vi "TestSuite_SQLiteOverallOperationCheck.vi"() -> ()   [LabVIEW 2014, in "TableLogger_SQLite_Actor.lvlib" / "TableLogger_SQLite_Actor.lvclass"]
uses:
  TableLogger_SQLite_Actor.lvclass
  TableLogger_Actor/TableLoggerConfig.ctl
  TableLogger_Actor/TableLoggerTypes.ctl
  TableLogger_Actor/TableLoggerBackupConfig.ctl
  <vilib>/addons/_JKI Toolkits/Caraya/classes/Test Suite/Test Suite.lvclass
  TableLogger_Actor/TableLogger_Actor.lvlib
panel:
  out "error out":errorcluster
  in  "error in (no error)":errorcluster
  # "Test Suite to Check overall operation of SQLite Logger"
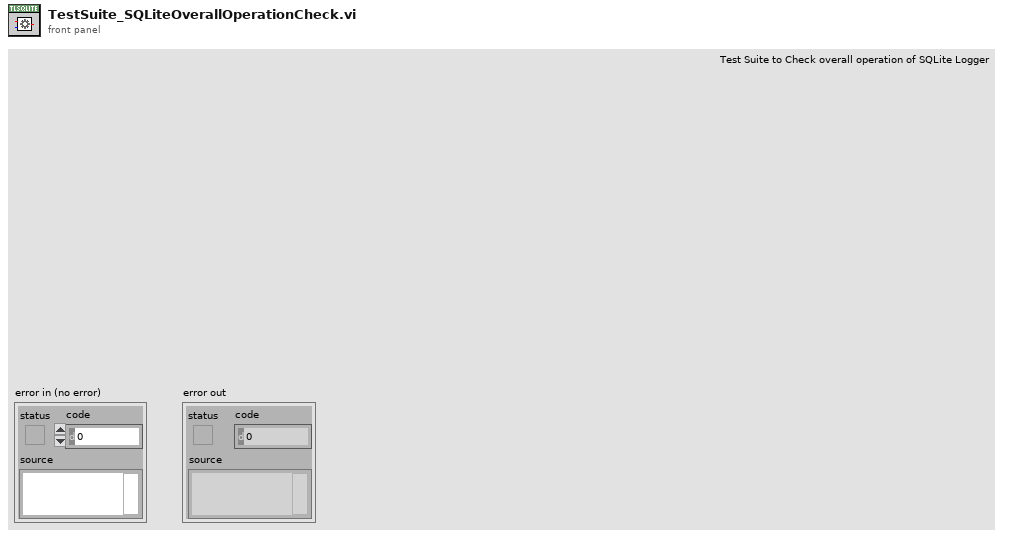
[diagram p1: front panel]
types:
  T1 = typedef "TableLogger_Actor.lvlib/TableLoggerConfig.ctl" = cluster{"TableLogger":T2, "DB File Path":path, "DB Backup Config":T3}
  T2 = typedef "TableLogger_Actor.lvlib/TableLoggerTypes.ctl" = enum16{"CSV Logger", "SQLite Logger"}
  T3 = typedef "TableLogger_Actor.lvlib/TableLoggerBackupConfig.ctl" = cluster{"Directory":path, "UTC Time Format":bool, "On Launch":bool, "Interval (Hours)":dbl, "Size Multiples (Bytes)":i32}
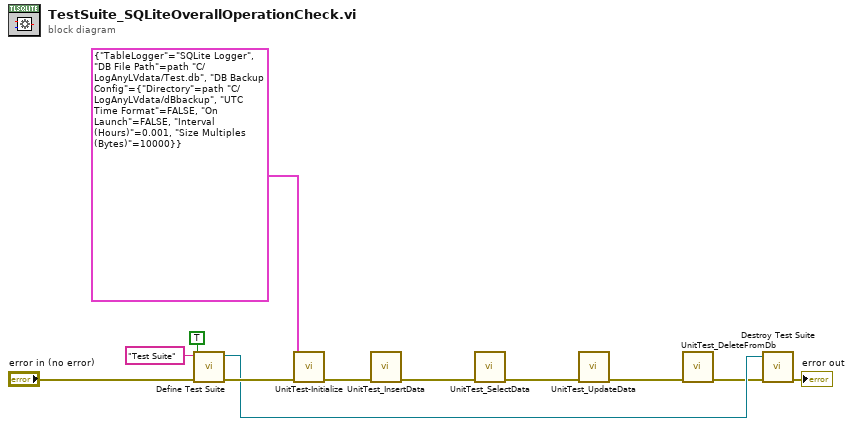
[diagram p0: block diagram]
diagram:
  n1 = call <vilib>:"Define Test Suite.vi"("error in (no error)"="error in (no error)", "Interactive"=TRUE, "Label (VI Title)"="Test Suite") -> ("error out"=w12:errorcluster, "Test Suite"=w9:refnum<class "Test Suite.lvclass">)  [unwired: 7 in]
  n2 = call "UnitTest-Initialize.vi"("error in"=w12, "Config IN"=T1 {"TableLogger"=enum."SQLite Logger", "DB File Path"=path "C:/LogAnyLVdata/Test.db", "DB Backup Config"={"Directory"=path "C:/LogAnyLVdata/dBbackup", "UTC Time Format"=FALSE, "On Launch"=FALSE, "Interval (Hours)"=0.001, "Size Multiples (Bytes)"=10000}} ("TableLogger Config")) -> ("error out"=w2:errorcluster)  [unwired: 7 in, 2 out]
  n3 = call "UnitTest_InsertData.vi"("error in (no error)"=w2) -> ("error out"=w5:errorcluster)  [unwired: 10 in]
  n4 = call "UnitTest_SelectData.vi"("error in (no error)"=w5) -> ("error out"=w4:errorcluster)  [unwired: 10 in]
  n5 = call "UnitTest_UpdateData.vi"("error in (no error)"=w4) -> ("error out"=w3:errorcluster)  [unwired: 10 in]
  n6 = call "UnitTest_DeleteFromDb.vi"("error in (no error)"=w3) -> ("error out"=w1:errorcluster)  [unwired: 10 in]
  n7 = call-dynamic "Destroy Test Suite.vi"("error in (no error)"=w1, "Test Suite in"=w9) -> ("error out"=→"error out":errorcluster)  [unwired: 9 in]
